vi "ILABs_RemoteCommandMgr.vi"(0 "action":string, 1 "data":string, 2 "appRef":refnum<vi>, 3 "viRef":refnum<vi>, 4 "errorIn":errorcluster) -> (5 "response":string, 7 "errorOut":string)   [LabVIEW 2009]
panel:
  out "Control":bool
  out "Connection Status":string
  in  "Case Constant\n(See Context Help)":bool=TRUE
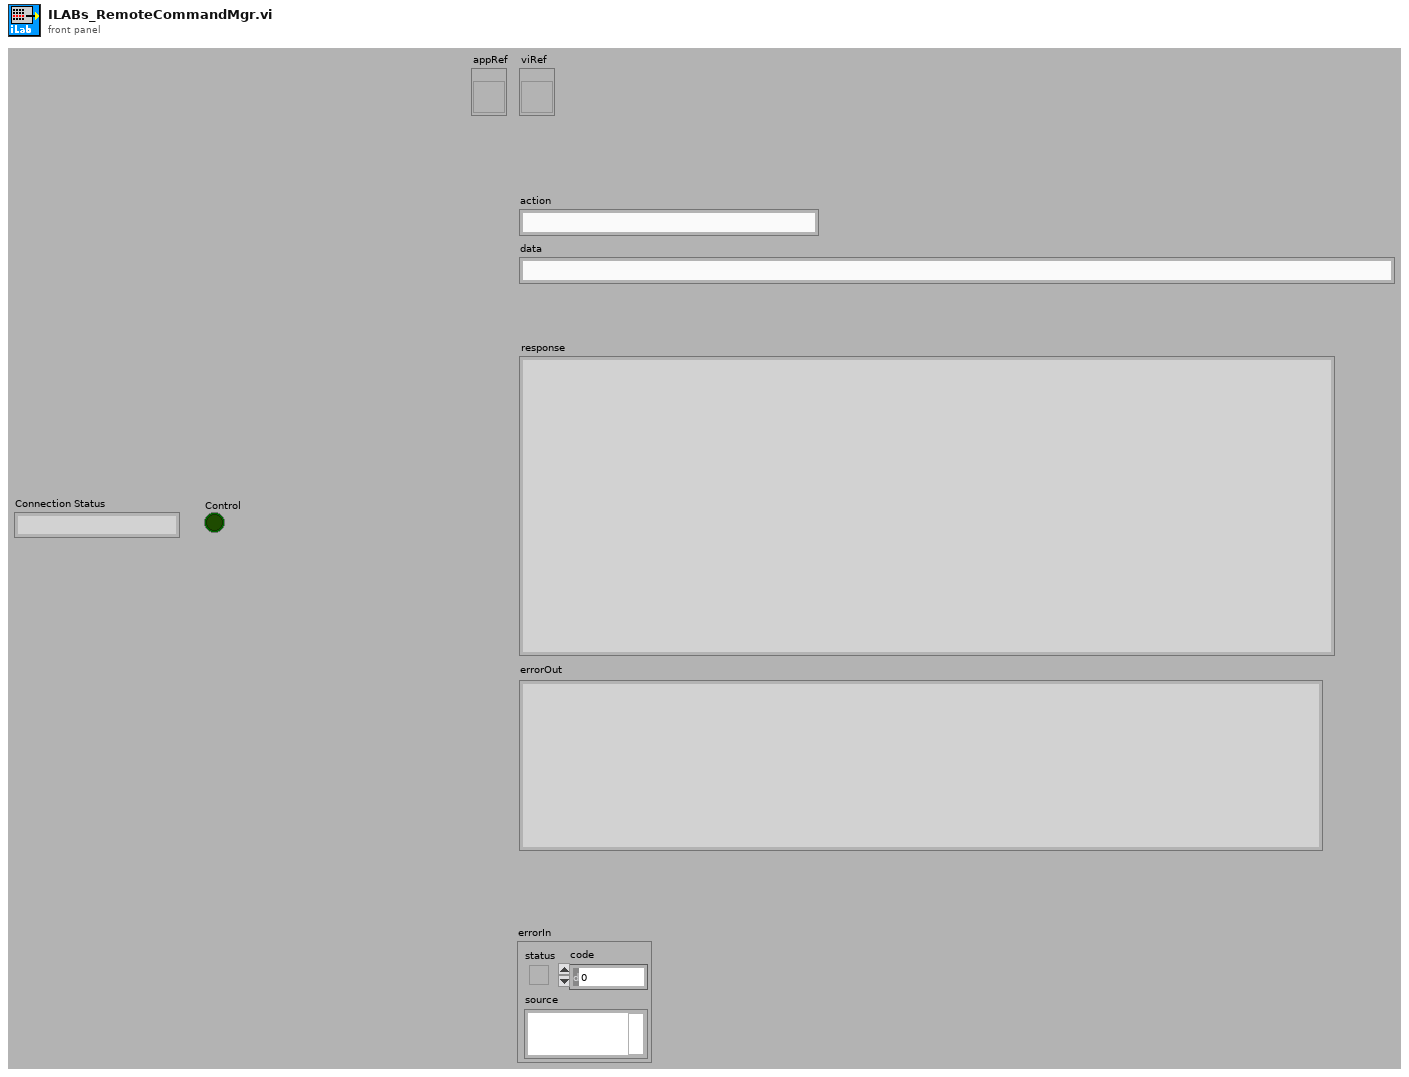
[diagram p1: front panel]
types:
  T1 = typedef "LVRemotePanelConnectionsTypeDef.ctl" = cluster{"VI Name":string, "Remote":string, "UserName":string, "Port":i32, "Status":enum32{"Viewing", "Waiting For Control", "Controlling"}, "Create Time":timestamp, "Status Time":timestamp, "Control End Time":timestamp}[]
  T2 = cluster{"VI Name":string, "Remote":string, "UserName":string, "Port":i32, "Status":enum32{"Viewing", "Waiting For Control", "Controlling"}, "Create Time":timestamp, "Status Time":timestamp, "Control End Time":timestamp}
  T3 = enum32{"Viewing", "Waiting For Control", "Controlling"}
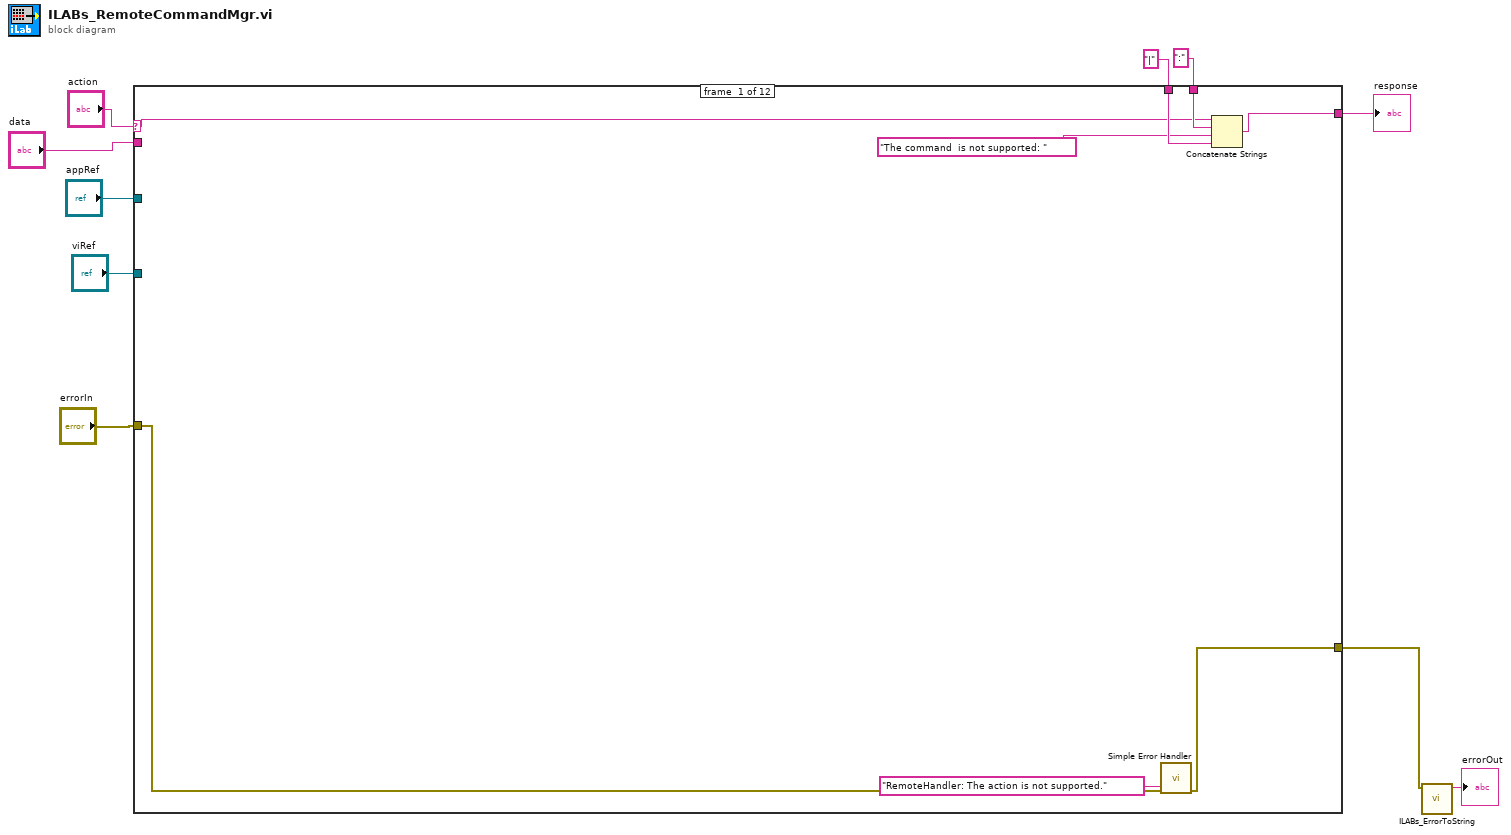
[diagram p0: block diagram]
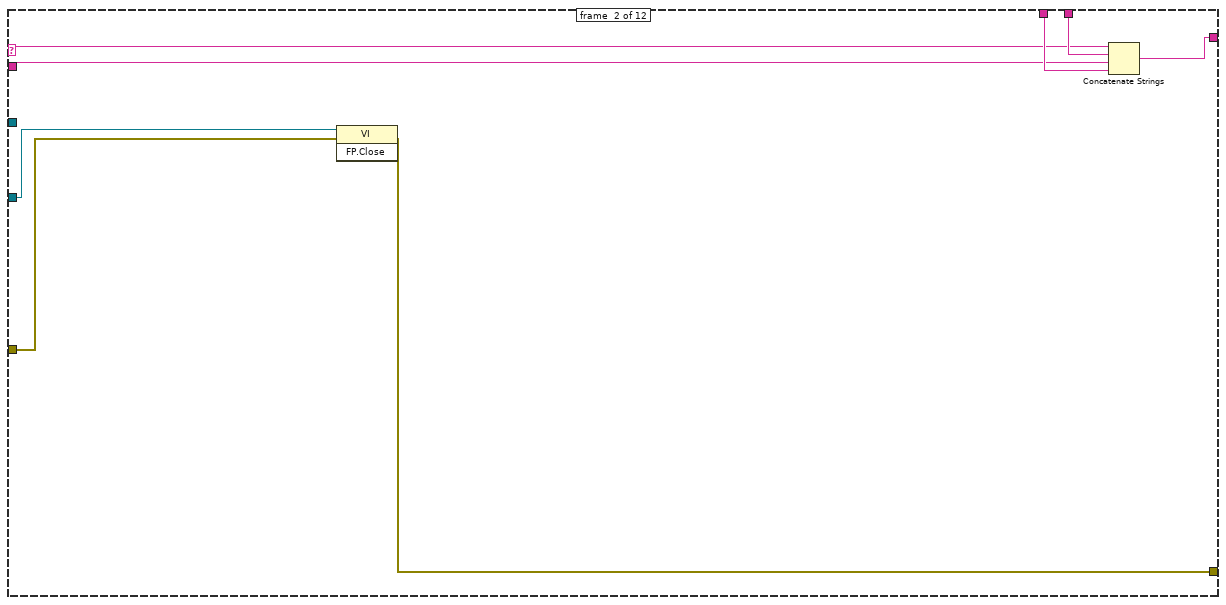
[diagram p2: hidden frame]
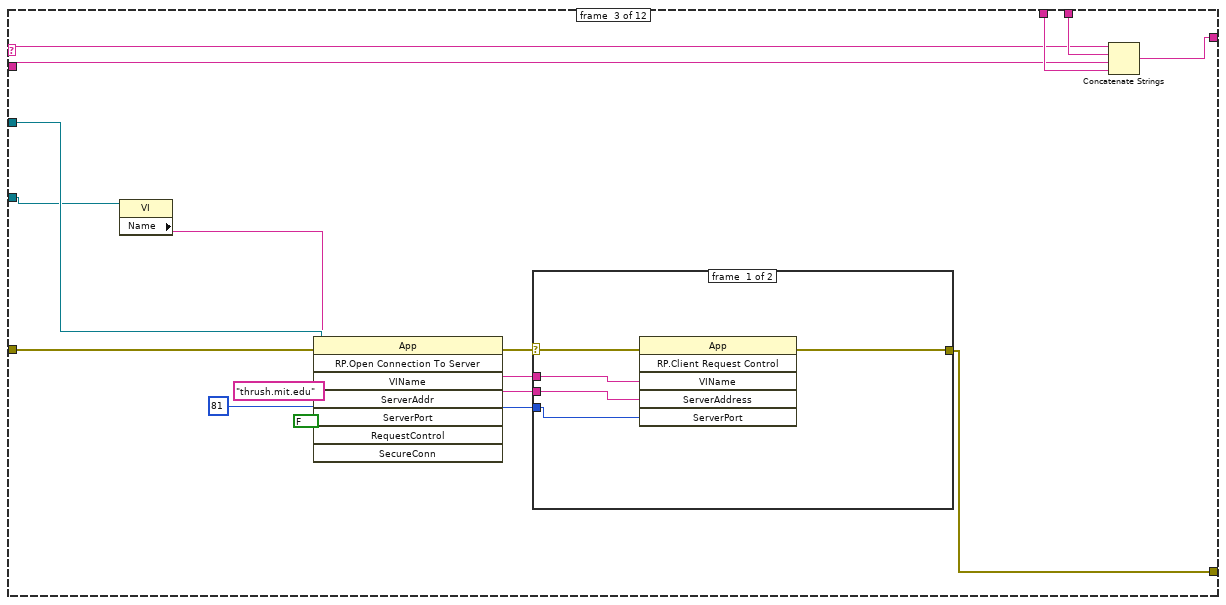
[diagram p3: hidden frame]
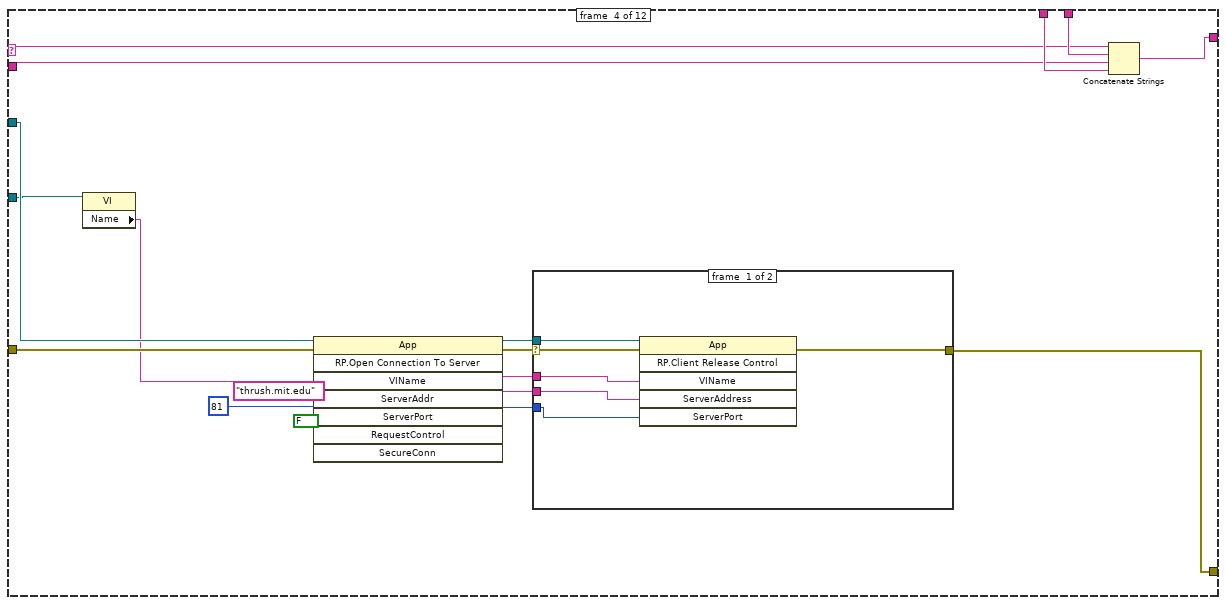
[diagram p5: hidden frame]
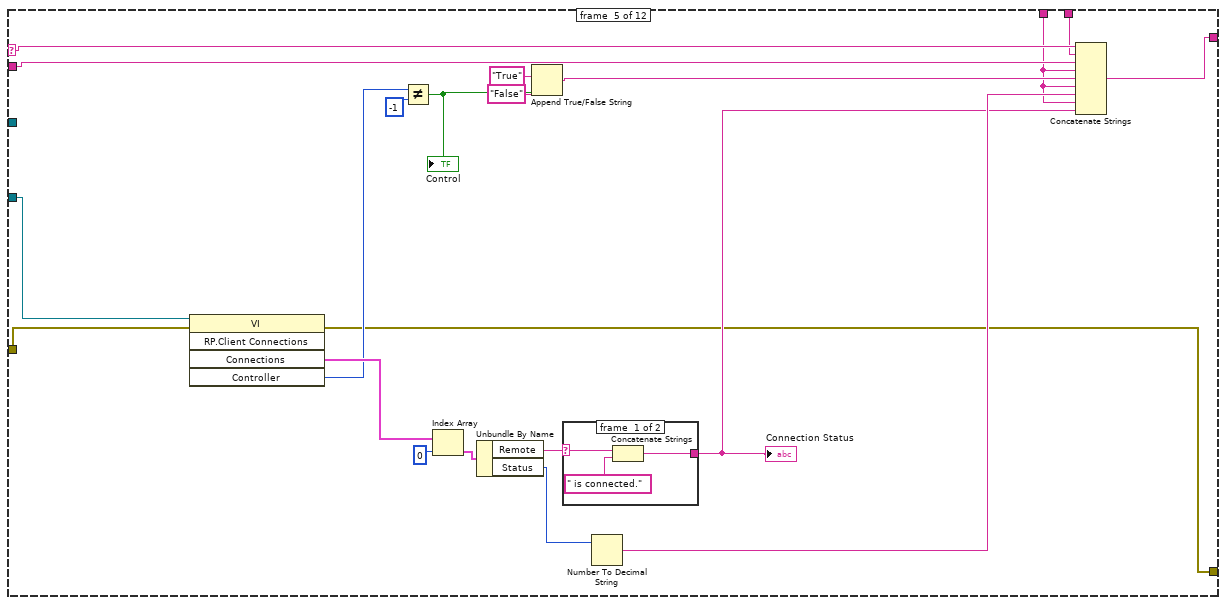
[diagram p7: hidden frame]
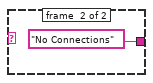
[diagram p8: hidden frame]
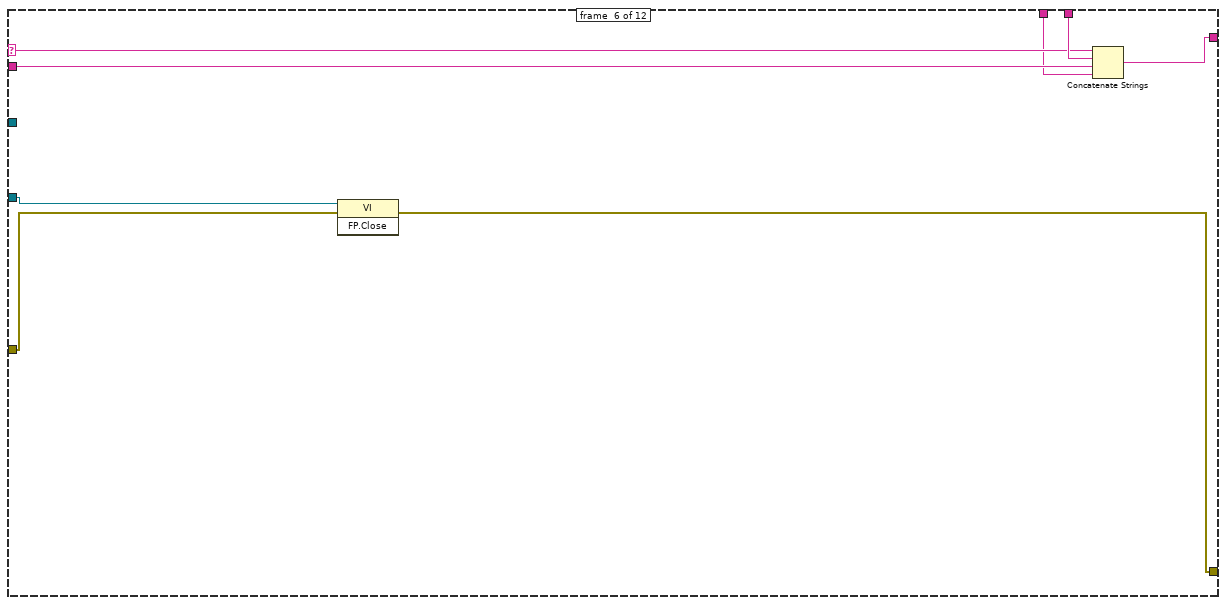
[diagram p9: hidden frame]
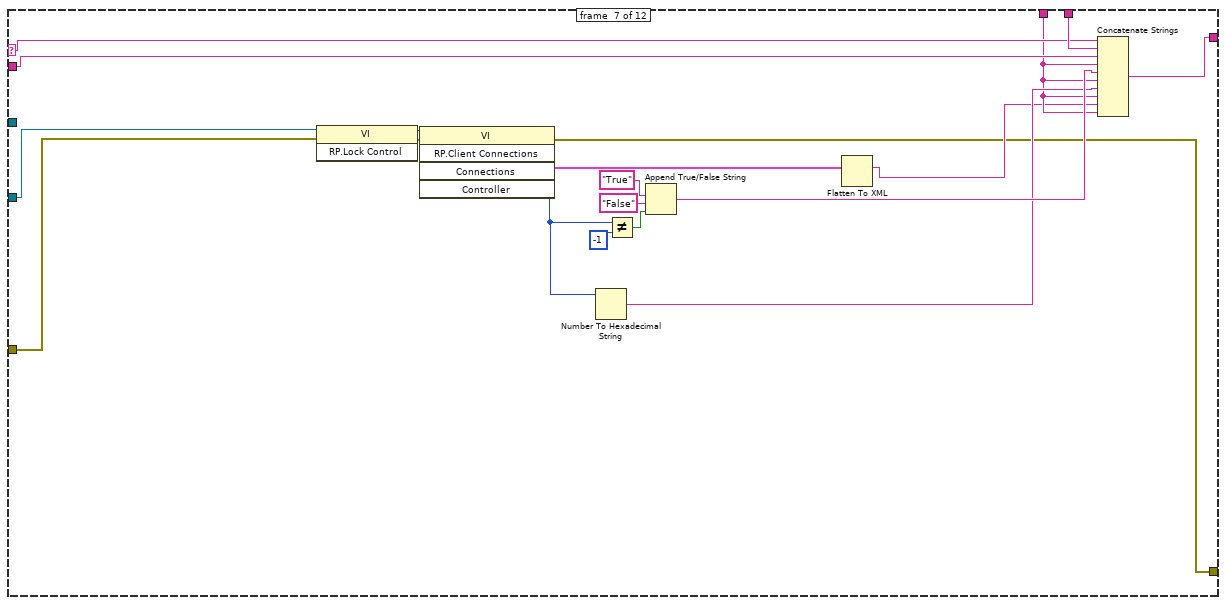
[diagram p10: hidden frame]
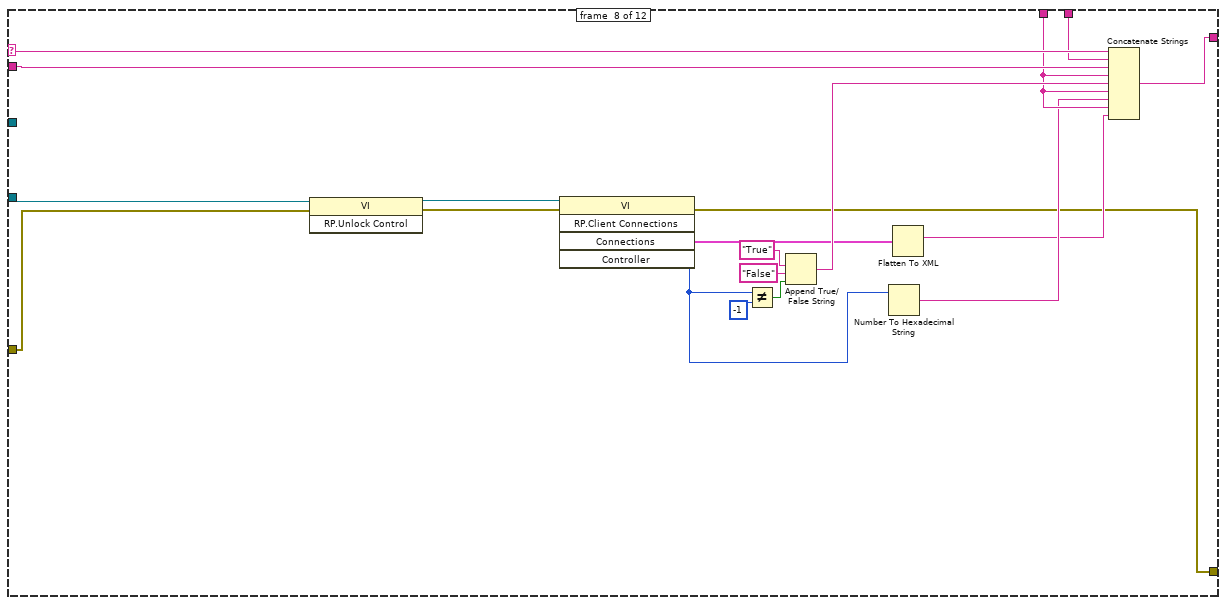
[diagram p11: hidden frame]
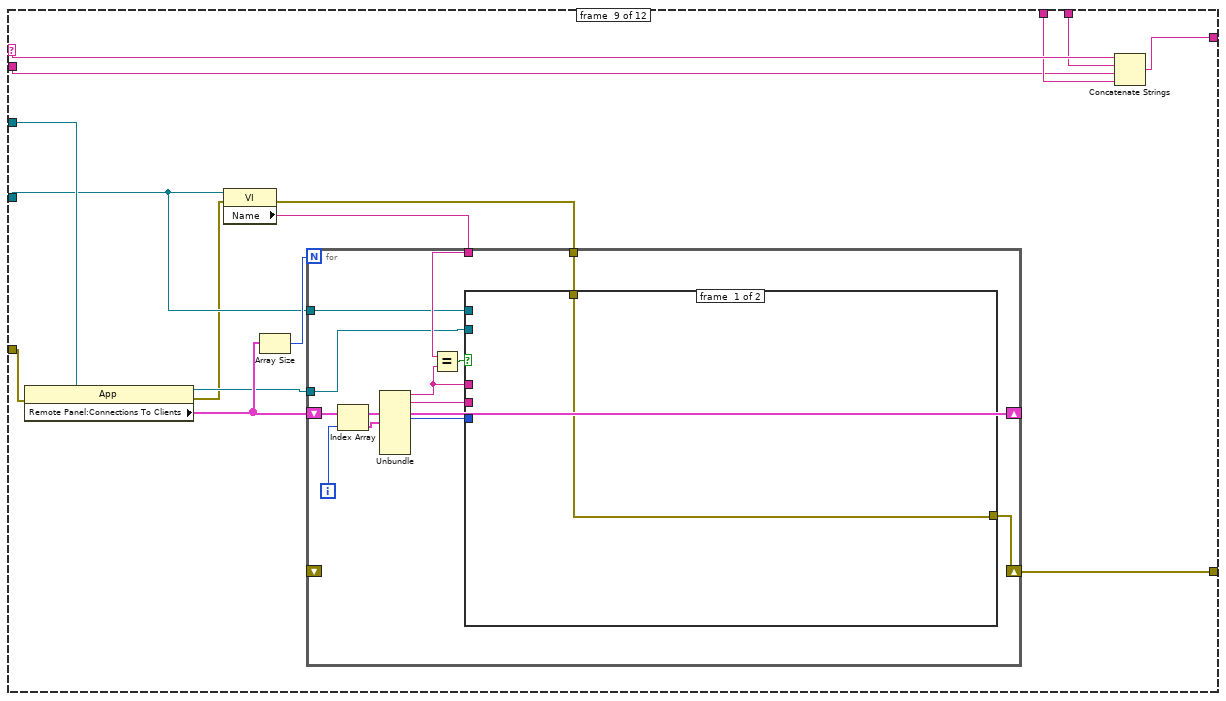
[diagram p12: hidden frame]
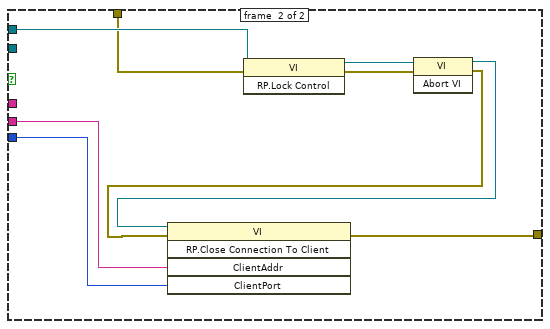
[diagram p13: hidden frame]
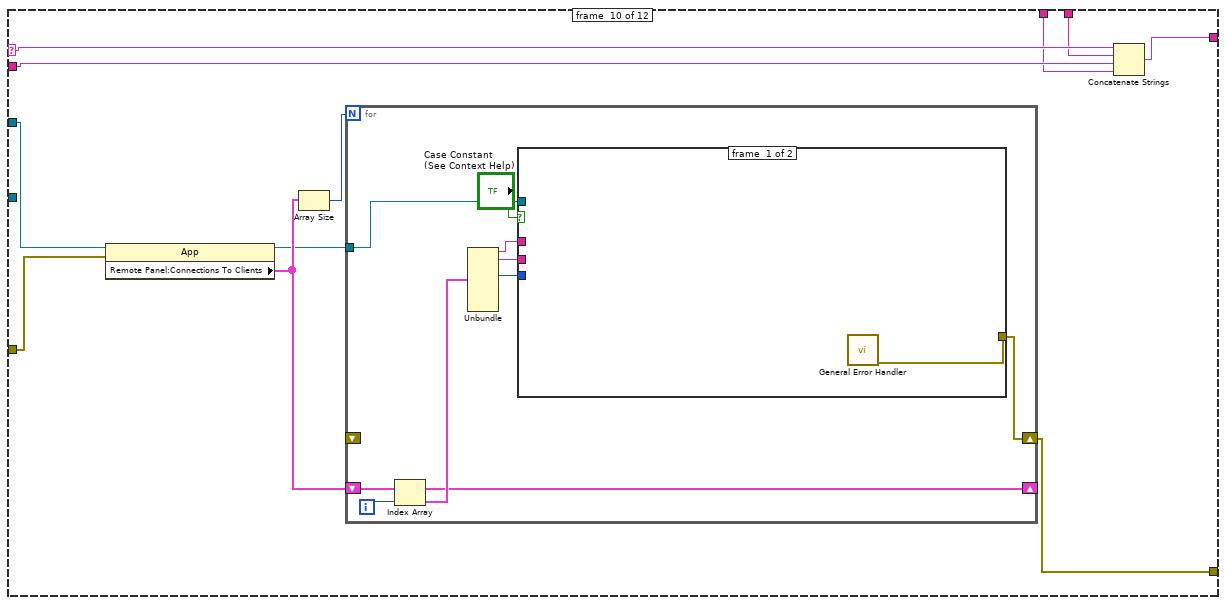
[diagram p14: hidden frame]
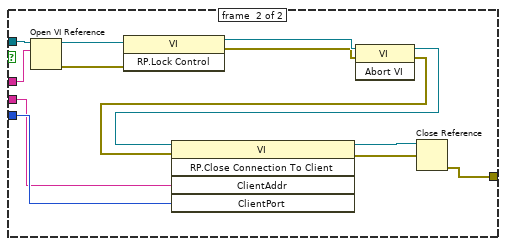
[diagram p15: hidden frame]
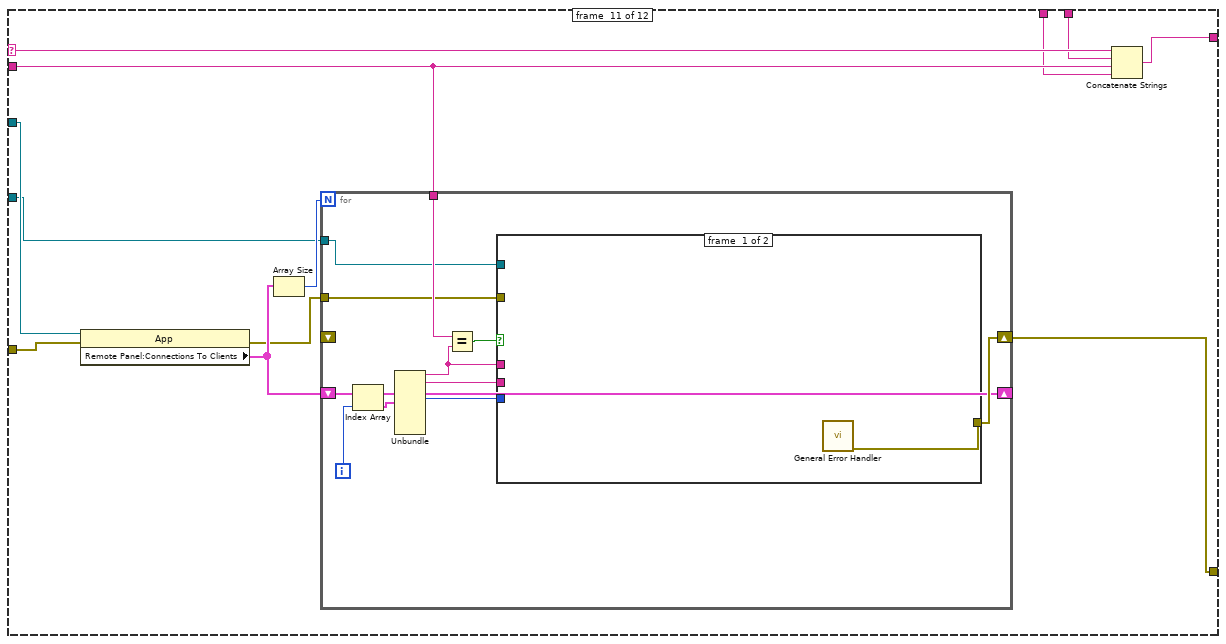
[diagram p16: hidden frame]
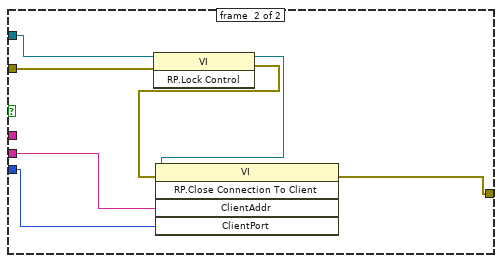
[diagram p17: hidden frame]
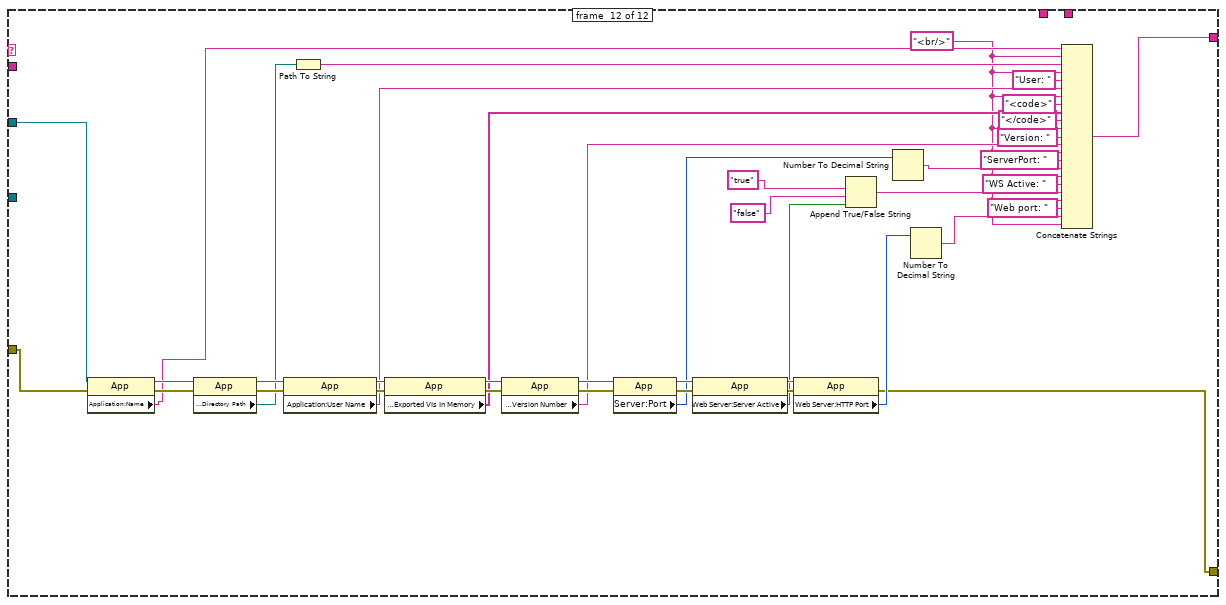
[diagram p18: hidden frame]
diagram:
  n1 = case shown="\"appStatus\"" "action" {
    selector: "action" -> [w13 w23 w37 w58 w77 w99 w112 w132 w149 w182 w218 _]
    tunnel: "data" -> [_ w22 w29 w53 w76 w98 w111 w131 w145 w181 w217 _]
    tunnel: [w18 w26 w40 w61 w89 w101 w120 w139 w154 w185 w222 w244] -> w9
    tunnel: "errorIn" -> [w11 w19 w32 w52 w71 w95 w103 w122 w150 w184 w219 w281]
    tunnel: ":" -> [w16 w24 w38 w59 w73 w100 w113 w130 w148 w180 w216 _]
    tunnel: "|" -> [w15 w25 w39 w60 w72 w97 w107 w128 w147 w179 w215 _]
    tunnel: "appRef" -> [_ _ w31 w51 _ _ _ _ w146 w178 w214 w243]
    tunnel: "viRef" -> [_ w20 w30 w50 w70 w96 w104 w123 w143 _ w213 _]
    tunnel: [w12 w21 w27 w47 w69 w94 w102 w121 w140 w177 w211 w242] -> w1
    frame #0 {
      (unwired) "The" ("message")
      n2 = call <vilib>:"Simple Error Handler.vi"("error source (\" \")"="RemoteHandler: The action is not supported." ("error source (\" \")"), "error in (no error)"=w11) -> ("error out"=w12:errorcluster)  [unwired: 1 in, 6 out]
      n3 = Concatenate Strings(w13, w16, "The command  is not supported: " ("string"), w15) -> (w18:string)
    }
    frame #1 {
      n4 = invoke class="VI" method="FP.Close"(reference=w20, error in=w19) -> (error out=w21:errorcluster)  [unwired: 1 in, 2 out]
      n5 = Concatenate Strings(w23, w24, w22, w25) -> (w26:string)
    }
    frame #2 {
      w34 = 81 ("Server Port")
      w35 = "thrush.mit.edu" ("Server Address")
      n6 = property class="VI"(reference=w30) -> ("Name"=w28:string)  [unwired: 1 in, 2 out]
      n7 = invoke class="App" method="RP.Open Connection To Server"(reference=w31, error in=w32, "VIName"=w28, "ServerAddr"=w35, "ServerPort"=w34, "RequestControl"=FALSE ("Request Control")) -> (error out=w33:errorcluster)  [unwired: 2 in, 7 out]
      n8 = case shown="No Error" w33 {
        selector: w33 -> [w45 w46]
        tunnel: w28 -> [w44 _]
        tunnel: w35 -> [w43 _]
        tunnel: w34 -> [w42 _]
        tunnel: [w41 w46] -> w27
        frame #0 {
          n9 = invoke class="App" method="RP.Client Request Control"(error in=w45, "VIName"=w44, "ServerAddress"=w43, "ServerPort"=w42) -> (error out=w41:errorcluster)  [unwired: 2 in, 5 out]
        }
        frame #1 {
        }
      }
      n10 = Concatenate Strings(w37, w38, w29, w39) -> (w40:string)
    }
    frame #3 {
      w55 = 81 ("Server Port")
      w56 = "thrush.mit.edu" ("Server Address")
      n11 = property class="VI"(reference=w50) -> ("Name"=w49:string)  [unwired: 1 in, 2 out]
      n12 = invoke class="App" method="RP.Open Connection To Server"(reference=w51, error in=w52, "VIName"=w49, "ServerAddr"=w56, "ServerPort"=w55, "RequestControl"=FALSE ("Request Control")) -> (reference out=w48:refnum<vi>, error out=w54:errorcluster)  [unwired: 2 in, 6 out]
      n13 = case shown="No Error" w54 {
        selector: w54 -> [w67 w68]
        tunnel: w49 -> [w66 _]
        tunnel: w56 -> [w65 _]
        tunnel: w55 -> [w64 _]
        tunnel: [w63 w68] -> w47
        tunnel: w48 -> [w62 _]
        frame #0 {
          n14 = invoke class="App" method="RP.Client Release Control"(reference=w62, error in=w67, "VIName"=w66, "ServerAddress"=w65, "ServerPort"=w64) -> (error out=w63:errorcluster)  [unwired: 1 in, 5 out]
        }
        frame #1 {
        }
      }
      n15 = Concatenate Strings(w58, w59, w53, w60) -> (w61:string)
    }
    frame #4 {
      n16 = invoke class="VI" method="RP.Client Connections"(reference=w70, error in=w71) -> (error out=w69:errorcluster, "Connections"=w88:T1, "Controller"=w85:i32)  [unwired: 3 in, 2 out]
      n17 = Not Equal?(x=w85, y=-1) -> (x != y?=w82:bool)
      "Control" <- w82
      n18 = Index Array(array=w88, index=0) -> (element=w83:T2)
      n19 = Unbundle By Name(w83) -> ("Remote"=w86:string, "Status"=w78:T3)
      n20 = Append True/False String(1:w82, 2:"False" ("false string"), 3:"True" ("true string")) -> (0:w79:string)  [unwired: 1 out]
      n21 = case shown="\"\"" w86 {
        selector: w86 -> [w92 _]
        tunnel: [w90 "No Connections"] -> w74
        frame #0 {
          n22 = Concatenate Strings(w92, " is connected." ("string")) -> (w90:string)
        }
        frame #1 {
        }
      }
      "Connection Status" <- w74
      n23 = Number To Decimal String(number=w78) -> (decimal integer string=w75:string)  [unwired: 1 out]
      n24 = Concatenate Strings(w77, w73, w76, w72, w79, w72, w75, w72, w74) -> (w89:string)
    }
    frame #5 {
      n25 = invoke class="VI" method="FP.Close"(reference=w96, error in=w95) -> (error out=w94:errorcluster)  [unwired: 1 in, 2 out]
      n26 = Concatenate Strings(w99, w100, w98, w97) -> (w101:string)
    }
    frame #6 {
      n27 = invoke class="VI" method="RP.Lock Control"(reference=w104, error in=w103) -> (reference out=w119:refnum<vi>, error out=w118:errorcluster)  [unwired: 1 in, 1 out]
      n28 = invoke class="VI" method="RP.Client Connections"(reference=w119, error in=w118) -> (error out=w102:errorcluster, "Connections"=w105:T1, "Controller"=w109:i32)  [unwired: 3 in, 2 out]
      n29 = Number To Hexadecimal String(2:w109) -> (0:w108:string)  [unwired: 1 out]
      n30 = Not Equal?(x=w109, y=-1) -> (x != y?=w116:bool)
      n31 = Append True/False String(1:w116, 2:"False" ("false string"), 3:"True" ("true string")) -> (0:w110:string)  [unwired: 1 out]
      n32 = Flatten To XML(anything=w105) -> (xml string=w106:string)
      n33 = Concatenate Strings(w112, w113, w111, w107, w110, w107, w108, w107, w106, w107) -> (w120:string)
    }
    frame #7 {
      n34 = invoke class="VI" method="RP.Unlock Control"(reference=w123, error in=w122) -> (reference out=w134:refnum<vi>, error out=w133:errorcluster)  [unwired: 1 in, 1 out]
      n35 = invoke class="VI" method="RP.Client Connections"(reference=w134, error in=w133) -> (error out=w121:errorcluster, "Connections"=w125:T1, "Controller"=w127:i32)  [unwired: 3 in, 2 out]
      n36 = Not Equal?(x=w127, y=-1) -> (x != y?=w137:bool)
      n37 = Append True/False String(1:w137, 2:"False" ("false string"), 3:"True" ("true string")) -> (0:w129:string)  [unwired: 1 out]
      n38 = Number To Hexadecimal String(2:w127) -> (0:w126:string)  [unwired: 1 out]
      n39 = Flatten To XML(anything=w125) -> (xml string=w124:string)
      n40 = Concatenate Strings(w132, w130, w131, w128, w129, w128, w126, w128, w124) -> (w139:string)
    }
    frame #8 {
      n41 = property class="App"(reference=w146, error in=w150) -> (reference out=w151:refnum<vi>, error out=w142:errorcluster, "Remote Panel:Connections To Clients"=w152:T1)
      n42 = property class="VI"(reference=w143, error in=w142) -> (error out=w141:errorcluster, "Name"=w144:string)  [unwired: 1 out]
      n43 = Array Size(array=w152) -> (size(s)=w153:i32)
      n44 = for {
        N: w153 -> [_]
        shift-right: [w159] -> _
        shift-left: w152 -> [w159]
        tunnel: w144 -> [w164]
        shift-right: [w155] -> w140
        shift-left: _ -> [_]
        tunnel: w151 -> [w158]
        tunnel: w143 -> [w157]
        tunnel: w141 -> [w156]
        i -> [w166]
        n45 = Index Array(array=w159, index=w166) -> (element=w165:T2)
        n46 = Unbundle(w165) -> ("VI Name"=w160:string, "Remote"=w161:string, "Port"=w162:i32)  [unwired: 5 out]
        n47 = Equal?(x=w164, y=w160) -> (x = y?=w163:bool)
        n48 = case shown="True" w163 {
          tunnel: w162 -> [_ w176]
          tunnel: w161 -> [_ w175]
          tunnel: w160 -> [_ _]
          tunnel: w158 -> [_ _]
          tunnel: w157 -> [_ w170]
          tunnel: w156 -> [w167 w169]
          tunnel: [w167 w168] -> w155
          frame #0 {
          }
          frame #1 {
            n49 = invoke class="VI" method="RP.Lock Control"(reference=w170, error in=w169) -> (reference out=w174:refnum<vi>, error out=w173:errorcluster)  [unwired: 1 in, 1 out]
            n50 = invoke class="VI" method="Abort VI"(reference=w174, error in=w173) -> (reference out=w171:refnum<vi>, error out=w172:errorcluster)  [unwired: 1 in, 1 out]
            n51 = invoke class="VI" method="RP.Close Connection To Client"(reference=w171, error in=w172, "ClientAddr"=w175, "ClientPort"=w176) -> (error out=w168:errorcluster)  [unwired: 1 in, 4 out]
          }
        }
      }
      n52 = Concatenate Strings(w149, w148, w145, w147) -> (w154:string)
    }
    frame #9 {
      n53 = property class="App"(reference=w178, error in=w184) -> (reference out=w183:refnum<vi>, "Remote Panel:Connections To Clients"=w186:T1)  [unwired: 1 out]
      n54 = Array Size(array=w186) -> (size(s)=w187:i32)
      n55 = for {
        N: w187 -> [_]
        shift-right: [w190] -> _
        shift-left: w186 -> [w190]
        shift-right: [w192] -> w177
        shift-left: _ -> [_]
        tunnel: w183 -> [w188]
        i -> [w196]
        n56 = Index Array(array=w190, index=w196) -> (element=w195:T2)
        n57 = Unbundle(w195) -> ("VI Name"=w191:string, "Remote"=w193:string, "Port"=w194:i32)  [unwired: 5 out]
        n58 = case shown="True" "Case Constant\n(See Context Help)" {
          tunnel: w194 -> [_ w210]
          tunnel: w193 -> [_ w209]
          tunnel: [w197 w208] -> w192
          tunnel: w191 -> [_ w207]
          tunnel: w188 -> [_ w198]
          frame #0 {
            n59 = call <vilib>:"General Error Handler.vi"() -> ("error out"=w197:errorcluster)  [unwired: 2 in, 13 out]
          }
          frame #1 {
            n60 = Open VI Reference(application reference (local)=w198, vi path=w207) -> (vi reference=w202:refnum<vi>, error out=w201:errorcluster)  [unwired: 1 in, 3 out]
            n61 = invoke class="VI" method="RP.Lock Control"(reference=w202, error in=w201) -> (reference out=w200:refnum<vi>, error out=w199:errorcluster)  [unwired: 1 in, 1 out]
            n62 = invoke class="VI" method="Abort VI"(reference=w200, error in=w199) -> (reference out=w203:refnum<vi>, error out=w204:errorcluster)  [unwired: 1 in, 1 out]
            n63 = invoke class="VI" method="RP.Close Connection To Client"(reference=w203, error in=w204, "ClientAddr"=w209, "ClientPort"=w210) -> (reference out=w206:refnum<vi>, error out=w205:errorcluster)  [unwired: 1 in, 3 out]
            n64 = Close Reference(reference=w206, error in (no error)=w205) -> (error out=w208:errorcluster)
          }
        }
      }
      n65 = Concatenate Strings(w182, w180, w181, w179) -> (w185:string)
    }
    frame #10 {
      n66 = property class="App"(reference=w214, error in=w219) -> (error out=w212:errorcluster, "Remote Panel:Connections To Clients"=w220:T1)  [unwired: 1 out]
      n67 = Array Size(array=w220) -> (size(s)=w221:i32)
      n68 = for {
        N: w221 -> [_]
        shift-right: [w226] -> _
        shift-left: w220 -> [w226]
        tunnel: w217 -> [w225]
        shift-right: [w228] -> w211
        shift-left: _ -> [_]
        tunnel: w213 -> [w224]
        tunnel: w212 -> [w223]
        i -> [w233]
        n69 = Index Array(array=w226, index=w233) -> (element=w232:T2)
        n70 = Unbundle(w232) -> ("VI Name"=w227:string, "Remote"=w229:string, "Port"=w230:i32)  [unwired: 5 out]
        n71 = Equal?(x=w225, y=w227) -> (x = y?=w231:bool)
        n72 = case shown="True" w231 {
          tunnel: w230 -> [_ w241]
          tunnel: w229 -> [_ w240]
          tunnel: [w234 w236] -> w228
          tunnel: w227 -> [_ _]
          tunnel: w224 -> [_ w237]
          tunnel: w223 -> [_ w235]
          frame #0 {
            n73 = call <vilib>:"General Error Handler.vi"() -> ("error out"=w234:errorcluster)  [unwired: 2 in, 13 out]
          }
          frame #1 {
            n74 = invoke class="VI" method="RP.Lock Control"(reference=w237, error in=w235) -> (reference out=w239:refnum<vi>, error out=w238:errorcluster)  [unwired: 1 in, 1 out]
            n75 = invoke class="VI" method="RP.Close Connection To Client"(reference=w239, error in=w238, "ClientAddr"=w240, "ClientPort"=w241) -> (error out=w236:errorcluster)  [unwired: 1 in, 4 out]
          }
        }
      }
      n76 = Concatenate Strings(w218, w216, w217, w215) -> (w222:string)
    }
    frame #11 {
      w245 = "<br/>" ("string")
      n77 = property class="App"(reference=w243, error in=w281) -> (reference out=w280:refnum<vi>, error out=w275:errorcluster, "Application:Name"=w266:string)
      n78 = property class="App"(reference=w280, error in=w275) -> (reference out=w279:refnum<vi>, error out=w274:errorcluster, "Application:Directory Path"=w264:path)
      n79 = property class="App"(reference=w279, error in=w274) -> (reference out=w278:refnum<vi>, error out=w273:errorcluster, "Application:User Name"=w262:string)
      n80 = Path To String(path=w264) -> (string=w265:string)
      n81 = property class="App"(reference=w278, error in=w273) -> (reference out=w277:refnum<vi>, error out=w272:errorcluster, "Application:Exported VIs In Memory"=w260:string[])
      n82 = property class="App"(reference=w277, error in=w272) -> (reference out=w276:refnum<vi>, error out=w271:errorcluster, "Application:Version Number"=w257:string)
      n83 = property class="App"(reference=w276, error in=w271) -> (reference out=w267:refnum<vi>, error out=w268:errorcluster, "Server:Port"=w254:u32)
      n84 = property class="App"(reference=w267, error in=w268) -> (reference out=w270:refnum<vi>, error out=w269:errorcluster, "Web Server:Server Active"=w252:bool)
      n85 = property class="App"(reference=w270, error in=w269) -> (error out=w242:errorcluster, "Web Server:HTTP Port"=w247:u16)  [unwired: 1 out]
      n86 = Append True/False String(1:w252, 2:"false" ("false string"), 3:"true" ("true string")) -> (0:w251:string)  [unwired: 1 out]
      n87 = Number To Decimal String(number=w254) -> (decimal integer string=w255:string)  [unwired: 1 out]
      n88 = Number To Decimal String(number=w247) -> (decimal integer string=w246:string)  [unwired: 1 out]
      n89 = Concatenate Strings(w266, w245, w265, w245, "User: " ("string"), w262, w245, "<code>" ("string"), w260, "</code>" ("string"), w245, "Version: " ("string"), w257, w245, "ServerPort: " ("string"), w255, w245, "WS Active: " ("string"), w251, w245, "Web port: " ("string"), w246, w245) -> (w244:string)
    }
  }
  "response" <- w9
  n90 = call "ILABs_ErrorToString.vi"("errorIn"=w1) -> ("errorOut"=→"errorOut":string)  [unwired: 10 out]
